vi "verify parameter in range.vi"(7 "parameter name":string, 8 "error in (no error)":errorcluster, 9 "lower limit":dbl format="%#_13g", 10 "value":dbl format="%#_13g", 11 "upper limit":dbl format="%#_13g") -> (0 "error out":errorcluster, 2 "verific error":errorcluster)   [LabVIEW 2018]
uses:
  <vilib>/ErrorRing/Error Ring.xnode
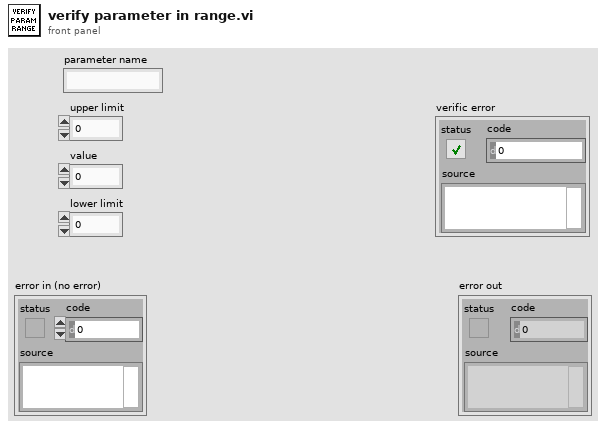
[diagram p1: front panel]
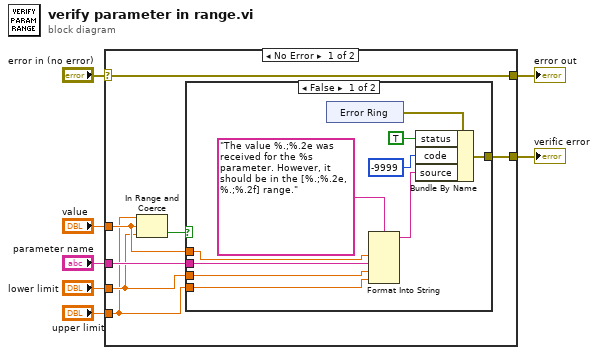
[diagram p0: block diagram]
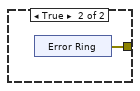
[diagram p2: hidden frame]
diagram:
  n1 = case shown="No Error" "error in (no error)" {
    selector: "error in (no error)" -> [w13 w28]
    tunnel: [w13 w28] -> w6
    tunnel: "lower limit" -> [w10 _]
    tunnel: "value" -> [w12 _]
    tunnel: "upper limit" -> [w9 _]
    tunnel: "parameter name" -> [w11 _]
    tunnel: [w8 _] -> w1
    frame No Error {
      n2 = In Range and Coerce(upper limit=w9, x=w12, lower limit=w10) -> (In Range?=w14:bool)  [unwired: 1 out]
      n3 = case shown="False" w14 {
        tunnel: w12 -> [w20 _]
        tunnel: w11 -> [w19 _]
        tunnel: w10 -> [w18 _]
        tunnel: w9 -> [w17 _]
        tunnel: [w16 w26] -> w8
        frame False {
          n4 = xnode "Error Ring"() -> ("error out"=w24:errorcluster)
          n5 = Format Into String(format string="The value %.;%.2e was received for the %s parameter. However, it should be in the [%.;%.2e, %.;%.2f] range." ("string"), w20, w19, w18, w17) -> (resulting string=w21:string)  [unwired: 2 in, 1 out]
          n6 = Bundle By Name(cluster=w24, "status"=TRUE, "code"=-9999, "source"=w21) -> (w16:errorcluster)
        }
        frame True {
          n7 = xnode "Error Ring"() -> ("error out"=w26:errorcluster)
        }
      }
    }
    frame Error {
    }
  }
  "error out" <- w6
  "verific error" <- w1
